vi "_Counter-Name.vi"(6 "LIBNAME":string, 8 "error in (no error)":errorcluster, 11 "StopSignal":T1) -> (0 "error out":errorcluster, 3 "name":string)   [LabVIEW 2017, in "StopSignal.lvlib"]
uses:
  StopSignal.lvlib
  Typedef/StopSignal.ctl
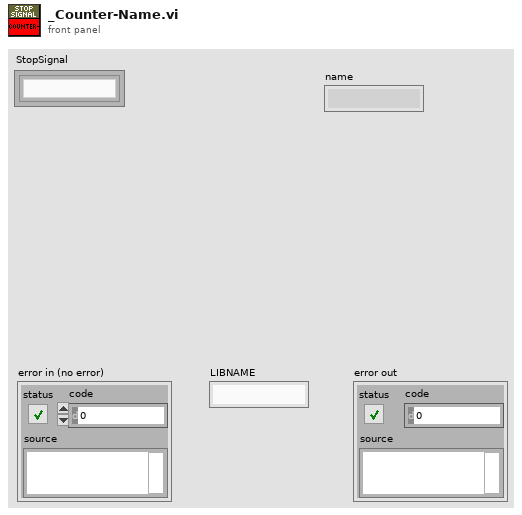
[diagram p1: front panel]
types:
  T1 = typedef "StopSignal.lvlib/StopSignal.ctl" = refnum<k1>
  T2 = cluster{"ObjMap":variant, "CntMap":variant, "SignalInArray":string[]}
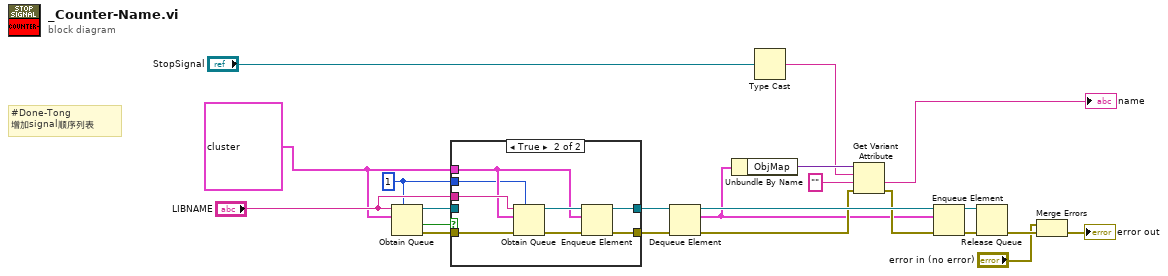
[diagram p0: block diagram]
diagram:
  w1 = T2 {"ObjMap"=variant, "CntMap"=variant, "SignalInArray"=[]}
  w10 = 1 ("max queue size (-1, unlimited)")
  # "#Done-Tong\n增加signal顺序列表"
  n1 = Obtain Queue(max queue size (-1, unlimited)=w10, name (unnamed)="LIBNAME", element data type=w1) -> (queue out=w19:refnum<queue>, created new?=w21:bool, error out=w20:errorcluster)  [unwired: 2 in]
  n2 = case shown="True" w21 {
    tunnel: w20 -> [w23 w30]
    tunnel: w19 -> [w24 _]
    tunnel: w1 -> [_ w26]
    tunnel: [w23 w32] -> w18
    tunnel: [w24 w31] -> w17
    tunnel: "LIBNAME" -> [_ w27]
    tunnel: w10 -> [_ w25]
    frame False {
    }
    frame True {
      n3 = Obtain Queue(max queue size (-1, unlimited)=w25, name (unnamed)=w27, element data type=w26, error in (no error)=w30) -> (queue out=w28:refnum<queue>, error out=w29:errorcluster)  [unwired: 1 in, 1 out]
      n4 = Enqueue Element(queue=w28, element=w26, error in (no error)=w29) -> (queue out=w31:refnum<queue>, error out=w32:errorcluster)  [unwired: 1 in, 1 out]
    }
  }
  n5 = Dequeue Element(queue=w17, error in (no error)=w18) -> (queue out=w16:refnum<queue>, element=w2:T2, error out=w4:errorcluster)  [unwired: 1 in, 1 out]
  n6 = Unbundle By Name(w2) -> ("ObjMap"=w9:variant)
  n7 = Type Cast(x="StopSignal") -> (*(type *) &x=w6:string)  [unwired: 1 in]
  n8 = Get Variant Attribute(Variant=w9, name=w6, default value (empty Variant)="" ("name(\"\")"), error in=w4) -> (value=→"name":string, error out=w3:errorcluster)  [unwired: 2 out]
  n9 = Enqueue Element(queue=w16, element=w2, error in (no error)=w3) -> (queue out=w15:refnum<queue>, error out=w14:errorcluster)  [unwired: 1 in, 1 out]
  n10 = Release Queue(queue=w15, error in (no error)=w14) -> (error out=w22:errorcluster)  [unwired: 1 in, 2 out]
  n11 = Merge Errors("error in (no error)", w22) -> (→"error out":errorcluster)
